vi "Enum Loop Complete.vi"(5 "Current State Enum":variant, 7 "Itteration":i32) -> (6 "# of Elements":i16, 8 "Loop Complete?":bool)   [LabVIEW 2015, in "Car Wash.lvlib" / "TLB`_Dependencies.lvlib"]
doc: "Is the Enum value last in series?\n\nUsed in simple Enum sequeneced state machines.\nTakes any enumeration and evaluates if the current value is the last in its series."
uses:
  TLB`_Dependencies.lvlib
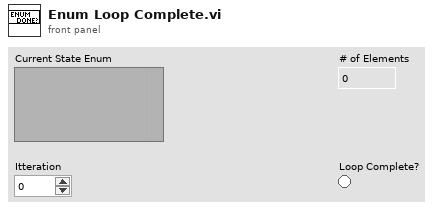
[diagram p1: front panel]
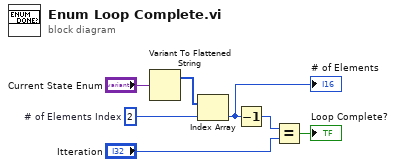
[diagram p0: block diagram]
diagram:
  w3 = 2  # # of Elements Index
  n1 = Variant To Flattened String(Variant="Current State Enum") -> (1:w2:i16[])  [unwired: 1 out]
  n2 = Index Array(array=w2, index=w3) -> (element=w4:i16)
  "# of Elements" <- w4
  n3 = Decrement(x=w4) -> (x-1=w1:i16)
  n4 = Equal?(x=w1, y="Itteration") -> (x = y?=→"Loop Complete?":bool)
